vi "AIM664 UDP Block Write.vi"() -> ()   [LabVIEW 2020]
uses:
  AIM664LV.lvlib
panel:
  in  "VL Control":T1={"VlId"=0, "SubVls"=2, "Bag"=16, "NetSelect"=3, "MaxFrameLength"=300, "FrameBufferSize"=300, "MACSourceLSLW"=563904, "MACSourceMSLW"=512, "Skew"=0} {"MACSourceMSLW" format="%.0x"; "NetSelect" items=["FDX_TX_FRAME_DLY_A"=0, "FDX_TX_FRAME_DLY_B"=1, "FDX_TX_FRAME_BOTH "=3, "FDX_TX_FRAME_ONLY_A"=4, "FDX_TX_FRAME_ONLY_B "=5]; "MACSourceLSLW" format="%.0x"}
  out "error out":errorcluster
  out "ResourceInfo 2":T2 {"PortMode" items=[" FDX_SINGLE", "FDX_REDUNDANT"]}
  out "ResourceInfo":T2 {"PortMode" items=[" FDX_SINGLE", "FDX_REDUNDANT"]}
  out "output cluster":T3={"GlobalResultCode"=0, "MsgCountOut"=2, "UdpBlockWriteResultArray"=[942640, 33, 0, 951280, 37, 0, 0, 0, 0, 0, 0, 0, 0, 0, 0, 0, 0, 0, 0, 0, 0, 0, 0, 0, 0, 0, 0, 0, 0, 0, 0, 0, 0, 0, 0, 0, 0, 0, 0, 0, 0, 0, 0, 0, 0, 0, 0, 0, 0, 0, 0, 0, 0, 0, 0, 0, 0, 0, 0, 0, 0, 0, 0, 0, 0, 0, 0, 0, 0, 0, 0, 0, 0, 0, 0, 0, 0, 0, 0, 0, 0, 0, 0, 0, 0, 0, 0, 0, 0, 0, 0, 0, 0, 0, 0, 0, 0, 0, 0, 0]}
  in  "Array 2":u32[](array[numeric])=[286331153, 572662306, 858993459, 1145324612, 1431655765, 1717986918, 2004318071, 2290649224, 2576980377, 170] format="%x"
  in  "Array":u32[](array[numeric])=[1985229328, 4275878552, 1985229328, 4275878552, 1985229328, 4275878552, 1985229328, 4275878552, 16] format="%x"
  in  "UDP Create Port2":T4={"PortType"=0, "UdpSrc"=2, "IpSrc"=167846145, "VlId"=0, "IpDst"=3772776448, "UdpDst"=2, "UdpNumBufMessages"=1, "UdpSamplingRate"=8, "UdpMaxMessageSize"=40, "SubVlId"=2} {"IpDst" format="%x"; "IpSrc" format="%x"}
  in  "UDP Create Port1":T4={"PortType"=0, "UdpSrc"=1, "IpSrc"=167846145, "VlId"=0, "IpDst"=3772776448, "UdpDst"=1, "UdpNumBufMessages"=1, "UdpSamplingRate"=8, "UdpMaxMessageSize"=40, "SubVlId"=1} {"IpDst" format="%x"; "IpSrc" format="%x"}
  in  "Input Cluster 2":T5 {"ExtendedStopMode" items=["FDX_ESTOP_NOT_USED", "FDX_ESTOP_EXT_TRG", "FDX_ESTOP_EXT_TRG_RESTART", "FDX_ESTOP_TIME"]; "StartMode" items=["FDX_STOP", "FDX_START", "FDX_START_TRG", "FDX_START_TIME"]}
  in  "Input Cluster":T5={"StartMode"=1, "Count"=100, "Sign"=0, "Day"=0, "Hour"=0, "Min"=0, "Second"=0, "MilliSec"=0, "MicroSec"=0, "ExtendedStopMode"=0, "TransmitTime"=0} {"ExtendedStopMode" items=["FDX_ESTOP_NOT_USED", "FDX_ESTOP_EXT_TRG", "FDX_ESTOP_EXT_TRG_RESTART", "FDX_ESTOP_TIME"]; "StartMode" items=["FDX_STOP", "FDX_START", "FDX_START_TRG", "FDX_START_TIME"]}
  in  "Input Cluster":T6={"SrvName"="local", "ClHostName"="local", "ClUser"="Brett", "ClApplication"="Test", "ClApplicationVersion"="V01.00", "ResourceID"=1, "Privileges"=4294967295} {"Privileges" items=["PRIVILEGES_ADMIN"=4294967295]}
  in  "Input Cluster":T7={"SrvName"="local", "ResourceID"=1, "ResourceType"=0} {"ResourceType" items=["Board", "Port"]}
  out "Output Cluster 2":T8={"ResourceID"=1, "ResourceType"=0, "ResourceInfo"="AMC-FDX-B2", "StructId"=0}
  in  "ServerRElement":u32=1
  in  "PortMap":u32=1
  out "Output Cluster":T9={"PortConfig"=0, "PortUsed"=1, "GlobalMemFree"=62889696, "SharedMemFree"=16566232} {"PortConfig" items=["FDX_SINGLE", "FDX_REDUNDANT"]}
  out "Output Cluster":T10={"Frames"=97, "TxStatus"=1, "TransmitMode"=2, "FramesPortB"=0} {"TransmitMode" items=["FDX_TX_GENERIC", "FDX_TX_REPLAY", "FDX_TX_INDIVIDUAL"]; "TxStatus" items=["FDX_STAT_STOP", "FDX_STAT_RUN", "FDX_STAT_ERROR", "FDX_STAT_WAIT_F_TRIG"]}
  in  "RerosPortDelay":u32
  in  "TransmitMode":u32(ring)=2 items=["FDX_TX_GENERIC", "FDX_TX_REPLAY", "FDX_TX_INDIVIDUAL"]
  in  "Input Cluster":T7={"SrvName"="local", "ResourceID"=2, "ResourceType"=1} {"ResourceType" items=["Board", "Port"]}
  in  "Input Cluster":T6={"SrvName"="local", "ClHostName"="local", "ClUser"="Brett", "ClApplication"="Test", "ClApplicationVersion"="V01.00", "ResourceID"=2, "Privileges"=4294967295} {"Privileges" items=["PRIVILEGES_ADMIN"=4294967295]}
  out "Output Cluster":T8={"ResourceID"=1, "ResourceType"=0, "ResourceInfo"="AMC-FDX-B2", "StructId"=0}
  in  "ServerRElement":u32=1
  out "NuOfResources":u32=3
  in  "SrvName":string="local"
  out "NuOfServers":u32=1
  # "ARINC 664 UDP Block Write"
  # "Overview: Configure the board to write UDP blocks into a Port.\nRequirement: At least one AIM ARINC-664 board with installed AIM ARINC 664 BSP.\nRestrictions: None.\nInstruction:\n1. Run the VI.\n2. Verify the results in the indicators."
  # "Tx Port"
  # "Board"
  # "Board"
  # "Tx Port"
  # "FdxTxPortInitCvi"
  # "FdxTxModeControlCvi"
  # "FdxTxCreateVLCvi"
  # "FdxTxUDPCreatePortCvi"
  # "FdxTxUDPCreatePortCvi"
  # "FdxLogoutCvi"
  # "FdxLogoutCvi"
  # "FdxTxControlCvi"
  # "FdxTxStatusCvi"
  # "FdxTxControlCvi"
  # "FdxTxUDPBlockWriteCvi"
  # "FdxInitCvi"
  # "CountServerResourcesCvi"
  # "GetServerResourcesCvi"
  # "QueryServerResourceCvi"
  # "FdxLoginCvi"
  # "GetServerResourcesCvi"
  # "QueryServerResourceCvi"
  # "FdxLoginCvi"
  # "Input"
  # "Input"
  # "Input"
  # "Input"
  # "Input"
  # "Input"
  # "Input"
  # "Input"
  # "Input"
  # "Input"
  # "Input"
  # "Input"
  # "Output"
  # "Input"
  # "Output"
  # "Output"
  # "Output"
  # "Output"
  # "Output"
  # "Output"
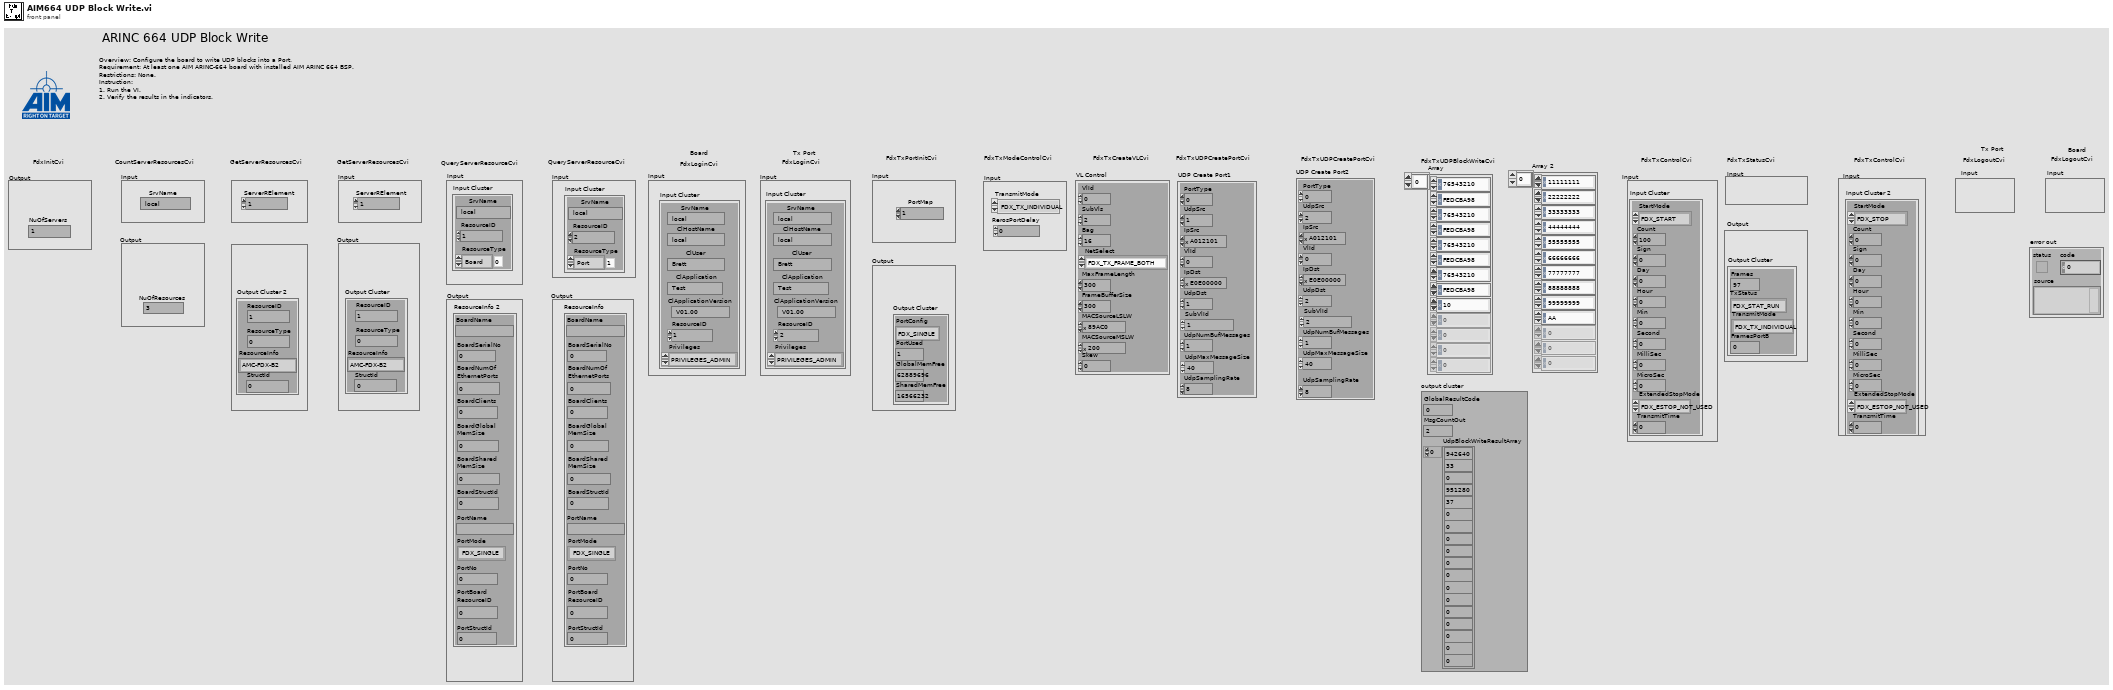
[diagram p1: front panel]
types:
  T1 = cluster{"VlId":u32, "SubVls":u32, "Bag":u32, "NetSelect":u32, "MaxFrameLength":u32, "FrameBufferSize":u32, "MACSourceLSLW":u32, "MACSourceMSLW":u32, "Skew":u32}
  T2 = cluster{"BoardName":string, "BoardSerialNo":u32, "BoardNumOf\nEthernetPorts":u32, "BoardClients":u32, "BoardGlobal\nMemSize":u32, "BoardShared\nMemSize":u32, "BoardStructId":u32, "PortName":string, "PortMode":u32, "PortNo":u32, "PortBoard\nResourceID":u32, "PortStructId":u32}
  T3 = cluster{"GlobalResultCode":i32, "MsgCountOut":u32, "UdpBlockWriteResultArray":u32[]}
  T4 = cluster{"PortType":u32, "UdpSrc":u32, "IpSrc":u32, "VlId":u32, "IpDst":u32, "UdpDst":u32, "UdpNumBufMessages":u32, "UdpSamplingRate":u32, "UdpMaxMessageSize":u32, "SubVlId":u32}
  T5 = cluster{"StartMode":i32, "Count":u32, "Sign":i32, "Day":u32, "Hour":u32, "Min":u32, "Second":u32, "MilliSec":u32, "MicroSec":u32, "ExtendedStopMode":i32, "TransmitTime":u32}
  T6 = cluster{"SrvName":string, "ClHostName":string, "ClUser":string, "ClApplication":string, "ClApplicationVersion":string, "ResourceID":u32, "Privileges":u32}
  T7 = cluster{"SrvName":string, "ResourceID":u32, "ResourceType":u32}
  T8 = cluster{"ResourceID":u32, "ResourceType":u32, "ResourceInfo":string, "StructId":u32}
  T9 = cluster{"PortConfig":u32, "PortUsed":u32, "GlobalMemFree":u32, "SharedMemFree":u32}
  T10 = cluster{"Frames":u32, "TxStatus":i32, "TransmitMode":u32, "FramesPortB":u32}
  T11 = cluster{"TxStatus":u32, "Frames":u32, "TransmitMode":u32, "FramesPortB":u32}
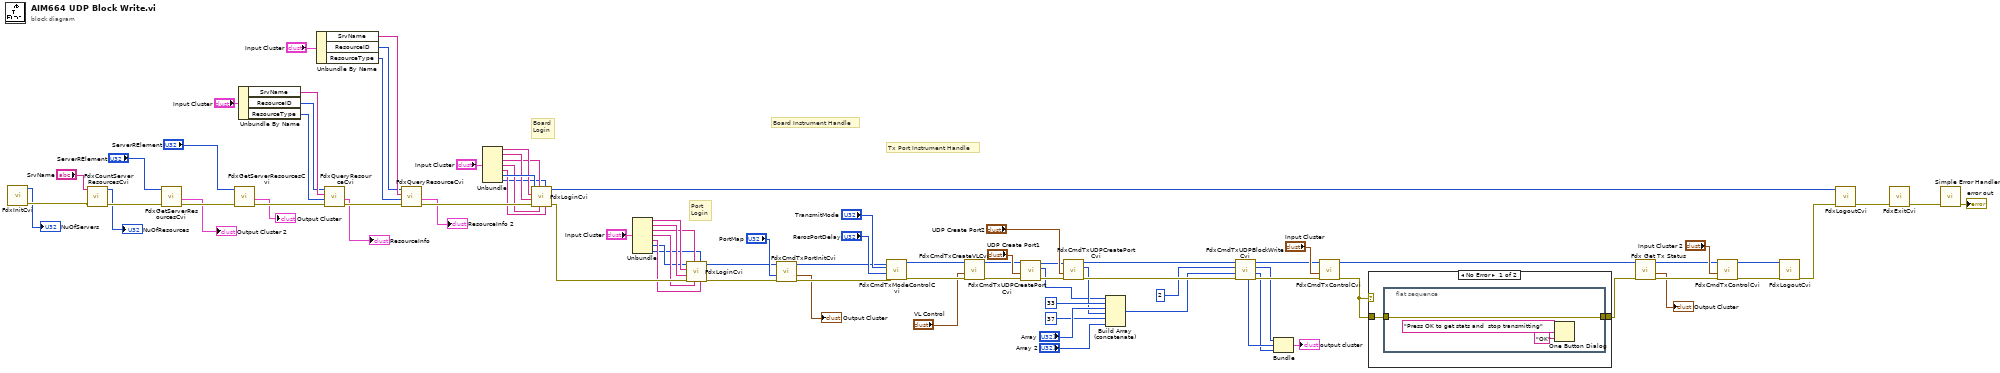
[diagram p0: block diagram]
diagram:
  # "Tx Port Instrument Handle"
  # "Board Instrument Handle"
  # "Port\nLogin"
  # "Board\nLogin"
  n1 = call "FdxInitCvi.vi"() -> ("error out"=w85:errorcluster, "Number of Servers"=→"NuOfServers":u32)  [unwired: 10 in]
  n2 = call "FdxCountServerResourcesCvi.vi"("error in"=w85, "SrvName (local)"="SrvName") -> ("error out"=w84:errorcluster, "Number of Resources"=→"NuOfResources":u32)  [unwired: 8 in]
  n3 = call "FdxGetServerResourcesCvi.vi"("error in"=w84, "ServerRElement"="ServerRElement") -> ("error out"=w83:errorcluster, "ServerResourceInfo"=→"Output Cluster 2":T8)  [unwired: 4 in, 4 out]
  n4 = call "FdxGetServerResourcesCvi.vi"("error in"=w83, "ServerRElement"="ServerRElement") -> ("error out"=w88:errorcluster, "ServerResourceInfo"=→"Output Cluster":T8)  [unwired: 4 in, 4 out]
  n5 = Unbundle By Name("Input Cluster") -> ("SrvName"=w38:string, "ResourceID"=w37:u32, "ResourceType"=w36:u32)
  n6 = Unbundle By Name("Input Cluster") -> ("SrvName"=w34:string, "ResourceID"=w33:u32, "ResourceType"=w32:u32)
  n7 = call "FdxQueryResourceCvi.vi"("error in"=w88, "ResourceType"=w36, "SrvName"=w38, "ResourceID"=w37) -> ("error out"=w82:errorcluster, "ResourceInfo"=→"ResourceInfo":T2)  [unwired: 5 in, 1 out]
  n8 = call "FdxQueryResourceCvi.vi"("error in"=w82, "ResourceType"=w32, "SrvName"=w34, "ResourceID"=w33) -> ("error out"=w81:errorcluster, "ResourceInfo"=→"ResourceInfo 2":T2)  [unwired: 5 in, 1 out]
  n9 = Unbundle("Input Cluster") -> ("SrvName"=w21:string, "ClHostName"=w20:string, "ClUser"=w19:string, "ClApplication"=w18:string, "ClApplicationVersion"=w17:string, "ResourceID"=w22:u32, "Privileges"=w16:u32)
  n10 = call "FdxLoginCvi.vi"("ClApplicationVersion"=w17, "Privileges"=w16, "ClApplication"=w18, "ClUser"=w19, "error in"=w81, "ClHostName"=w20, "SrvName"=w21, "ResourceID"=w22) -> ("error out"=w80:errorcluster, "InstrumentHandle"=w50:u32)  [unwired: 2 in]
  n11 = Unbundle("Input Cluster") -> ("SrvName"=w30:string, "ClHostName"=w29:string, "ClUser"=w28:string, "ClApplication"=w27:string, "ClApplicationVersion"=w26:string, "ResourceID"=w25:u32, "Privileges"=w24:u32)
  n12 = call "FdxLoginCvi.vi"("ClApplicationVersion"=w26, "Privileges"=w24, "ClApplication"=w27, "ClUser"=w28, "error in"=w80, "ClHostName"=w29, "SrvName"=w30, "ResourceID"=w25) -> ("error out"=w71:errorcluster, "InstrumentHandle"=w43:u32)  [unwired: 2 in]
  n13 = call "FdxCmdTxPortInitCvi.vi"("error in"=w71, "PortMap"="PortMap", "InstrumentHandle_port"=w43) -> ("error out"=w87:errorcluster, "PortInitOut"=→"Output Cluster":T9, "InstrumentHandle_port"=w49:u32)  [unwired: 6 in]
  n14 = call "FdxCmdTxModeControlCvi.vi"("error in"=w87, "RerosPortDelay"="RerosPortDelay", "TransmitMode"="TransmitMode", "InstrumentHandle_port"=w49) -> ("error out"=w76:errorcluster, "InstrumentHandle_port"=w48:u32)  [unwired: 6 in]
  n15 = call "FdxCmdTxCreateVLCvi.vi"("error in"=w76, "Input Cluster"="VL Control", "InstrumentHandle_port in"=w48) -> ("error out"=w75:errorcluster, "InstrumentHandle_port out"=w47:u32)  [unwired: 7 in]
  n16 = call "FdxCmdTxUDPCreatePortCvi.vi"("error in"=w75, "UdpDescription"="UDP Create Port1", "InstrumentHandle"=w47) -> ("error out"=w74:errorcluster, "UdpHandle"=w5:u32, "InstrumentHandle"=w46:u32)  [unwired: 6 in]
  n17 = call "FdxCmdTxUDPCreatePortCvi.vi"("error in"=w74, "UdpDescription"="UDP Create Port2", "InstrumentHandle"=w46) -> ("error out"=w72:errorcluster, "UdpHandle"=w12:u32, "InstrumentHandle"=w45:u32)  [unwired: 6 in]
  n18 = Build Array (concatenate)(w5, u32 33 ("element"), "Array", w12, u32 37 ("element"), "Array 2") -> (w6:u32[])
  n19 = call "FdxCmdTxUDPBlockWriteCvi.vi"("error in"=w72, "UdpBlockWriteMsgArray"=w6, "MsgCount"=u32 2, "InstrumentHandle"=w45) -> ("error out"=w73:errorcluster, "UdpBlockWriteResultArray"=w8:u32[], "GlobalResultCode"=w10:i32, "InstrumentHandle"=w44:u32, "MsgCountOut"=w9:u32)  [unwired: 3 in]
  n20 = Bundle("GlobalResultCode"=w10, "MsgCountOut"=w9, "UdpBlockWriteResultArray"=w8) -> (→"output cluster":T3)  [unwired: 1 in]
  n21 = call "FdxCmdTxControlCvi.vi"("error in"=w73, "TxControl"="Input Cluster", "InstrumentHandle_port in"=w44) -> ("error out"=w2:errorcluster, "InstrumentHandle_port out"=w42:u32)  [unwired: 7 in]
  n22 = case shown="No Error" w2 {
    tunnel: w2 -> [w90 w94]
    tunnel: [w89 w94] -> w86
    frame No Error {
      n23 = flat-sequence {
        tunnel: w90 -> [w93]
        tunnel: [w93] -> w89
        frame #0 {
          n24 = One Button Dialog(message="Press OK to get stats and  stop transmitting", button name ("OK")="OK") -> ()  [unwired: 1 out]
        }
      }
    }
    frame Error {
    }
  }
  n25 = call "Fdx Get Tx Status.vi"("error in"=w86, "InstrumentHandle_port"=w42) -> ("error out"=w79:errorcluster, "TxStatus"=→"Output Cluster":T11, "InstrumentHandle_port"=w41:u32)  [unwired: 7 in]
  n26 = call "FdxCmdTxControlCvi.vi"("error in"=w79, "TxControl"="Input Cluster 2", "InstrumentHandle_port in"=w41) -> ("error out"=w77:errorcluster, "InstrumentHandle_port out"=w40:u32)  [unwired: 7 in]
  n27 = call "FdxLogoutCvi.vi"("error in"=w77, "InstrumentHandle"=w40) -> ("error out"=w78:errorcluster)  [unwired: 9 in]
  n28 = call "FdxLogoutCvi.vi"("error in"=w78, "InstrumentHandle"=w50) -> ("error out"=w70:errorcluster)  [unwired: 9 in]
  n29 = call "FdxExitCvi.vi"("error in"=w70) -> ("error out"=w4:errorcluster)  [unwired: 10 in]
  n30 = call <vilib>:"Simple Error Handler.vi"("error in (no error)"=w4) -> ("error out"=→"error out":errorcluster)  [unwired: 4 in, 4 out]
